vi "SplitDMAFIFOData.vi"(8 "error in (no error)":errorcluster, 10 "Save Illumination Mask?":bool, 11 "Data Array IN":u64[](array[numeric])) -> (0 "error out":errorcluster, 1 "Image trig index":u16[](array[numeric]), 2 "Time at P_final if less than t_final":u32[](array[numeric]), 3 "Final step, n":u16[](array[numeric]))   [LabVIEW 2016]
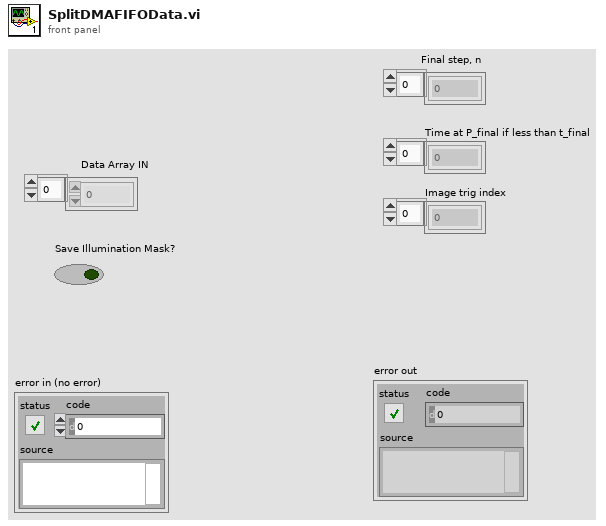
[diagram p1: front panel]
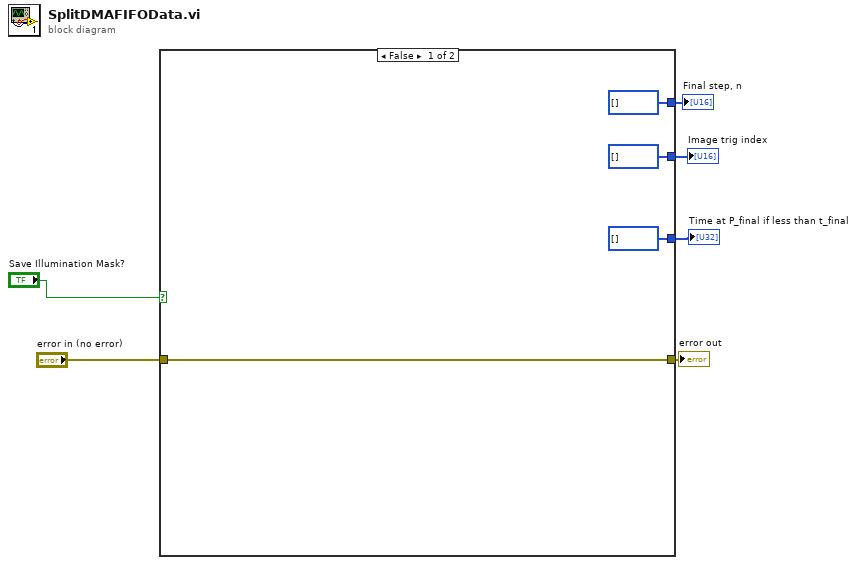
[diagram p0: block diagram]
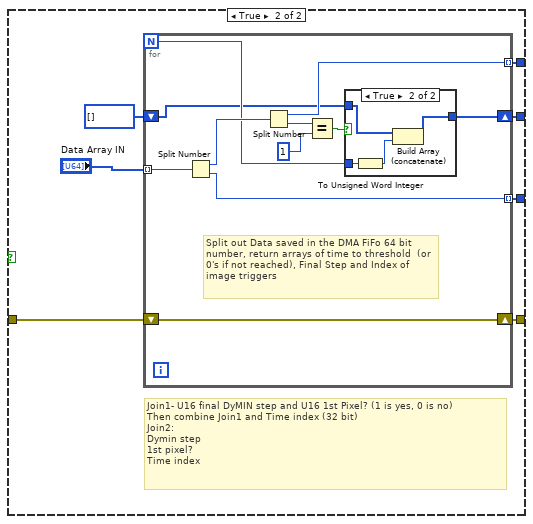
[diagram p2: hidden frame]
diagram:
  n1 = case shown="False" "Save Illumination Mask?" {
    tunnel: [w8 w17] -> w6
    tunnel: [u32[] [] w15] -> w5
    tunnel: [u16[] [] w14] -> w4
    tunnel: "error in (no error)" -> [w8 w12]
    tunnel: [u16[] [] w11] -> w1
    frame False {
    }
    frame True {
      # "Join1- U16 final DyMIN step and U16 1st Pixel? (1 is yes, 0 is no)\nThen combine Join1 and Time index (32 bit)\nJoin2:\nDymin step\n1st pixel?\nTime index"
      n2 = for {
        N -> [w20]
        tunnel: "Data Array IN" -> [w27] mode=indexing
        shift-right: [w28] -> w17
        shift-left: w12 -> [w28]
        tunnel: [w26] -> w15 mode=indexing
        tunnel: [w24] -> w14 mode=indexing
        shift-right: [w19] -> w11
        shift-left: u16[] [] -> [w18]
        # "Split out Data saved in the DMA FiFo 64 bit number, return arrays of time to threshold  (or 0's if not reached), Final Step and Index of image triggers"
        n3 = Split Number(x=w27) -> (hi(x)=w25:u32, lo(x)=w26:u32)
        n4 = Split Number(x=w25) -> (hi(x)=w24:u16, lo(x)=w23:u16)
        n5 = Equal?(x=w23, y=u16 1) -> (x = y?=w21:bool)
        n6 = case shown="True" w21 {
          tunnel: w20 -> [_ w31]
          tunnel: w18 -> [w29 w33]
          tunnel: [w29 w32] -> w19
          frame False {
          }
          frame True {
            n7 = To Unsigned Word Integer(number=w31) -> (unsigned 16bit integer=w30:u16)
            n8 = Build Array (concatenate)(w33, w30) -> (w32:u16[])
          }
        }
      }
    }
  }
  "error out" <- w6
  "Time at P_final if less than t_final" <- w5
  "Final step, n" <- w4
  "Image trig index" <- w1
